vi "ConvertStrMacAddrToByteMacAddr.vi"(11 "eMacAddr":string="02:00:00:20:00:00") -> (3 "ByteMacAddr":u8[](array[numeric]) format="%02x")   [LabVIEW 2018, in "Library-DataConvert.lvlib"]
uses:
  Library-DataConvert.lvlib
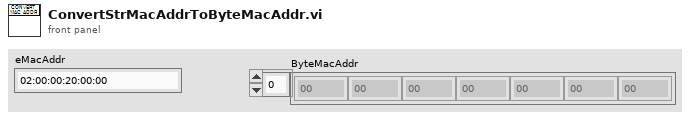
[diagram p1: front panel]
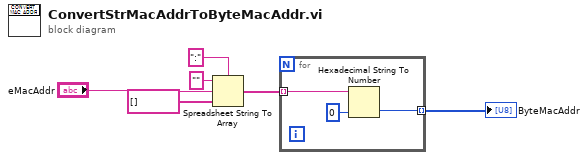
[diagram p0: block diagram]
diagram:
  n1 = Spreadsheet String To Array(delimiter (Tab)=":" ("구분 문자 (탭)"), format string="" ("포맷 문자열"), spreadsheet string="eMacAddr", array type (2D Dbl)=string[] []) -> (array=w2:string[])
  n2 = for {
    tunnel: w2 -> [w9] mode=indexing
    tunnel: [w7] -> w1 mode=indexing
    n3 = Hexadecimal String To Number(string=w9, default (0uL)=u8 0 ("기본(0 U32)")) -> (number=w7:u8)  [unwired: 1 in, 1 out]
  }
  "ByteMacAddr" <- w1
